vi "ReadLakeshoreSettings (SubVI).vi"(5 "Prepended command":string, 6 "error in (no error)":errorcluster, 8 "Channel Str":string, 9 "Lakeshore port":refnum<visa-resource-name>) -> (0 "error out":errorcluster, 2 "Settings array out":i32[](array[numeric]), 3 "VISA Refnum out":refnum<visa-resource-name>)   [LabVIEW 2017, in "Fridge Software v2.1.lvlib"]
uses:
  Fridge Software v2.1.lvlib
  <instrlib>/Lake Shore 372/Lake Shore 372.lvlib
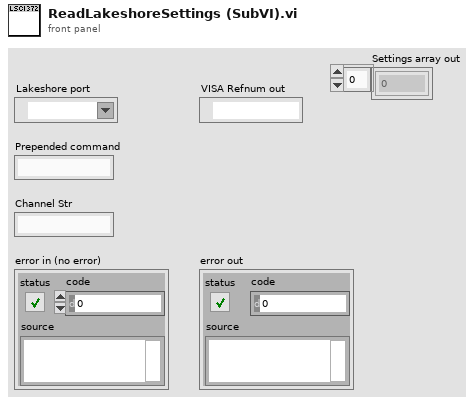
[diagram p1: front panel]
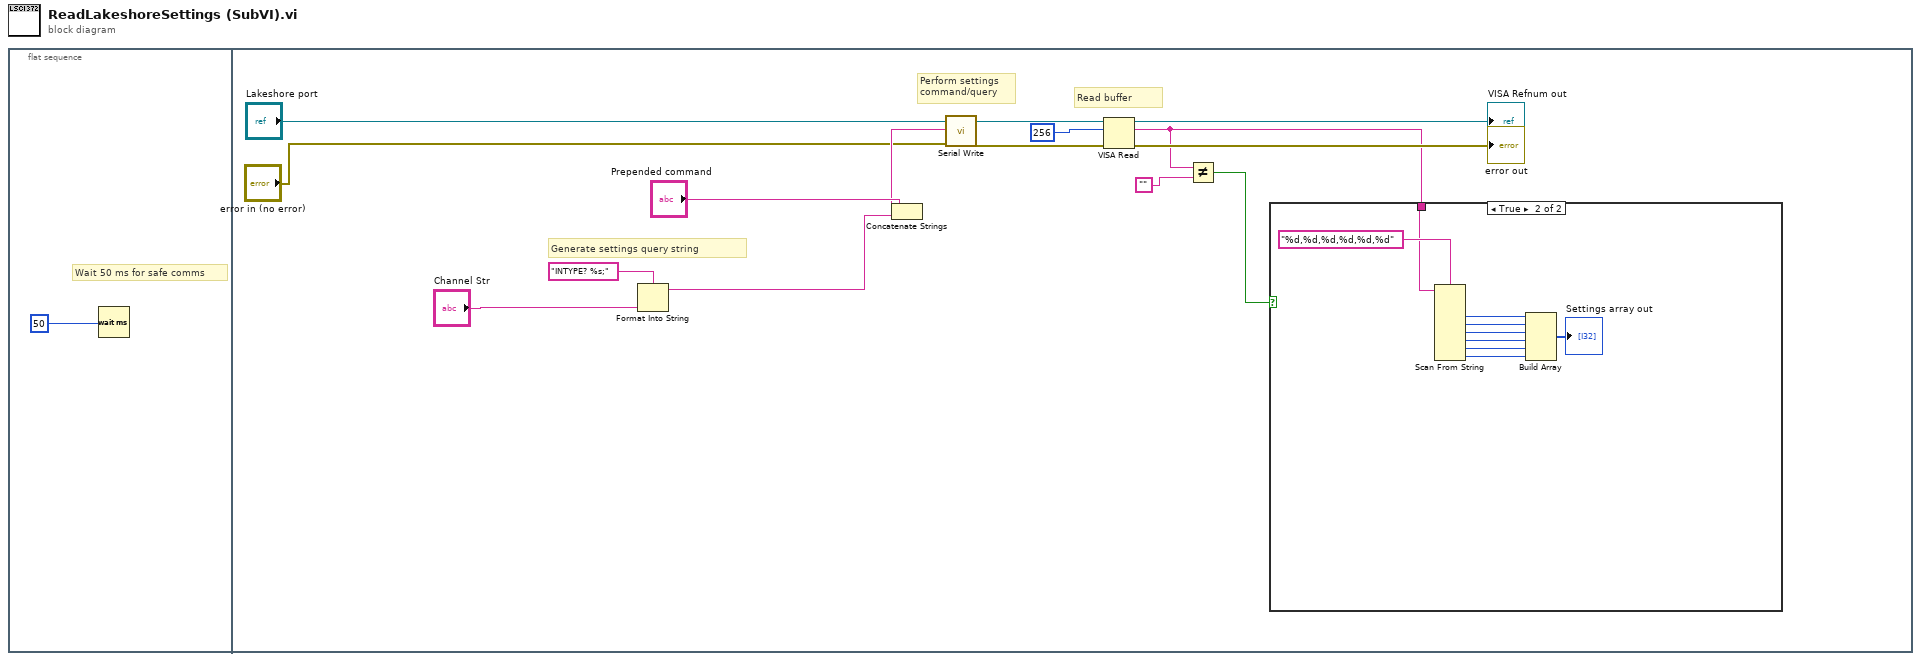
[diagram p0: block diagram]
diagram:
  n1 = flat-sequence {
    frame #0 {
      # "Wait 50 ms for safe comms"
      n2 = Wait (ms)(milliseconds to wait=50) -> ()  [unwired: 1 out]
    }
    frame #1 {
      # "Generate settings query string"
      # "Read buffer"
      # "Perform settings command/query"
      n3 = Format Into String(format string="INTYPE? %s;", "Channel Str") -> (resulting string=w12:string)  [unwired: 2 in, 1 out]
      n4 = Concatenate Strings("Prepended command", w12) -> (w8:string)
      n5 = call <instrlib>:"Serial Write.vi"("error in (no error)"="error in (no error)", "Write Buffer (\"\")"=w8, "VISA resource name"="Lakeshore port") -> ("error out"=w5:errorcluster, "VISA resource name out"=w6:refnum<visa-resource-name>)  [unwired: 6 in, 1 out]
      n6 = VISA Read(VISA resource name=w6, byte count=u32 256, error in (no error)=w5) -> (VISA resource name out=→"VISA Refnum out":refnum<visa-resource-name>, read buffer=w3:string, error out=→"error out":errorcluster)  [unwired: 1 out]
      n7 = Not Equal?(x=w3, y="") -> (x != y?=w2:bool)
      n8 = case shown="True" w2 {
        tunnel: w3 -> [_ w19]
        frame False {
        }
        frame True {
          n9 = Scan From String(format string="%d,%d,%d,%d,%d,%d", input string=w19) -> (output 1=w21:i32, output 2=w22:i32, output 3=w23:i32, output 4=w24:i32, output 5=w25:i32, output 6=w17:i32)  [unwired: 8 in, 3 out]
          n10 = Build Array(w21, w22, w23, w24, w25, w17) -> (→"Settings array out":i32[])
        }
      }
    }
  }
